vi "FFT Co-processor (FPGA) 6592R.vi"() -> ()   [LabVIEW 2014]
doc: "Data From Host Loop:\nThe FPGA target recieves a signal from the host from the Host-to-FPGA DMA FIFO and stores that data in the FIFO IN target-scoped FIFO. FIFO IN will not be written to if there is no information being read from the host and the Host-to-FPGA FIFO has timed out. The loop will stop if the user presses the stop control button or if the FIFO IN times out and data transfer from the host to the target is complete.\n\nFFT Processing Loop:\nWhen the FFT Express VI has signaled that it is ready for input, it will begin to read data from the FIFO IN target-scoped FIFO. The user has control over the output of the FFT Express VI. As the FFT VI computes the FFT it writes the resulting data to the FIFO OUT target-scoped VI when the FFT output is valid. The loop will stop if the user presses the stop control button or if the FIFO OUT times out and data transfer from the FFT VI to the FIFO is complete.\n\nData To Host Loop:\nFIFO OUT transfers data back to the host by writing the computed FFT signal data to the FPGA-to-Host DMA FIFO. When there is no data in FIFO OUT, it times out and stops writing to the host. At this point the data transfer is complete."
uses:
  <vilib>/Platform/TimedLoop/XDataNode/timing_clust.ctl
  <vilib>/Platform/TimedLoop/XDataNode/nitl_modes.ctl
  <vilib>/Platform/TimedLoop/XDataNode/wakeup.ctl
  <vilib>/rvi/Analysis/measure/FFT/simModelSupport/niFPGA FFT Streaming Sim Properties.ctl
  <vilib>/rvi/Analysis/measure/FFT/simModelSupport/niFPGA FFT Sim Stream Group Properties.ctl
  <vilib>/rvi/Analysis/measure/FFT/simModelSupport/niFPGA FFT Sim Types.ctl
  <vilib>/rvi/Analysis/measure/FFT/simModelSupport/niFpgaFFTSimArithmeticProperties.ctl
  <vilib>/rvi/Analysis/measure/FFT/simModelSupport/niFpgaFFTSimDfxp.ctl
  <vilib>/fxp/LVFixedPointQuantizationPolicyTypeDef.ctl
  <vilib>/rvi/Analysis/measure/FFT/XNode/niFpgaFFTButterflyDelays.ctl
  <vilib>/rvi/Analysis/measure/FFT/simModelSupport/niFPGA FFT Sim Properties.ctl
  <vilib>/rvi/Emulation/niFpgaSctlEmulationGetInTimedLoop.vi
  <vilib>/rvi/Emulation/niFpgaEmulationReportErrorSimple.vi
  <vilib>/rvi/Emulation/niFpgaGetClockAttributes.vi
  <vilib>/rvi/Emulation/niFpgaCriticalErrorInLSC.vi
  <vilib>/rvi/Emulation/niFpgaProcessEmulError.vi
  <vilib>/rvi/Emulation/niFpgaEmulationIsFPGAContextNoSignature.vi
  <vilib>/rvi/errors/niFpgaSetErrorForExecOnDevCompSimple.vi
  <vilib>/rvi/eio/common/nirviEmuReportErrorAndStop.vi
  <vilib>/rvi/DataTransferAndStorage/Container/Common/niFpgaContainerGetUniqueNameForEmu.vi
  <vilib>/rvi/FIFO/Fifo_Resource/nirvififoEmulationSetSize.vi
  <vilib>/rvi/FIFO/Fifo_Resource/nirviFifoEmulationQueueMgr.vi
  <instcachedir>/0/nirviFifoEmulationQueueMgr_E5CAEC123FF24DC58D834DCA3CDAA9B5.lvgen/nirviFifoEmulationQueueMgr_E5CAEC123FF24DC58D834DCA3CDAA9B5_002.vi
  <vilib>/Utility/error.llb/Clear Errors.vi
  <vilib>/rvi/FIFO/Fifo_Resource/nirvififoEmulationCreateLock.vi
  <vilib>/rvi/FIFO/Fifo_Resource/nirvififoEmulationObtainLock.vi
  <vilib>/rvi/FIFO/Fifo_Resource/nirvififoEmulationReleaseLock.vi
  <vilib>/rvi/occurrence/nirviWaitOnOccurrenceBase.vi
  <vilib>/rvi/errors/nirviReportUnexpectedCaseInternalError.vi
  <vilib>/rvi/errors/nirviReportUnexpectedCaseInternalError (U32).vi
  <vilib>/rvi/Analysis/measure/FFT/simModelSupport/niFpgaFFTSimModelStreamingCore.vi
  <vilib>/rvi/Analysis/measure/FFT/simModelSupport/niFpgaFFTSimModelCore.vi
  <vilib>/rvi/FIFO/Fifo_Resource/nirvififoEmulationDetermineInputValidOut.vi
  <vilib>/rvi/interface/RandomDataEmulation/niFpgaRandomDataHandleErrors.vi
  <vilib>/Platform/TimedLoop/XDataNode/XDataNode.xnode
  <vilib>/rvi/DataTransferAndStorage/Container/XNode/niFpgaContainer.xnode
  <vilib>/rvi/FIFO/Fifo_Resource/nirvififoEmulationRead.vi
  <vilib>/rvi/Analysis/measure/FFT/XNode/niFpgaFFT.xnode
  <vilib>/rvi/FIFO/Fifo_Resource/nirvififoEmulationWrite.vi
  <vilib>/rvi/interface/RandomDataEmulation/nirviRandomDataFpgaReadWriteTemplate.vi
  <vilib>/Platform/TimedLoop/XDataNode/XDNodeRunTimeDep.lvlib
panel:
  in  "FFT Size":i16=8192
  out "FFT Out":i32
  out "FIFO In (loop 2)":i32
  out "FIFO In":i32
  out "Host to FPGA":i32
  in  "stop":bool
  # "This FPGA VI continuously receives data from the host, performs a 1 kByte FFT, and then transfers the FFT results back to the host.  The input data type for the FFT is a 16-bit fixed point number with 8 bits of integer precision."
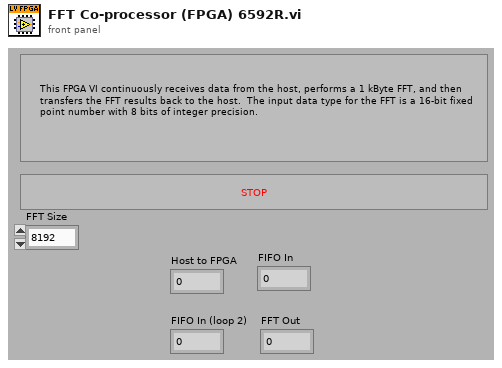
[diagram p1: front panel]
types:
  T1 = typedef "XDNodeRunTimeDep.lvlib/timing_clust.ctl" = cluster{"Expected End [f-1]":u64, "Actual End [f-1]":u64, "Finished Late? [f-1]":bool, "Expected End [i-1]":u64, "Actual End [i-1]":u64, "Finished Late? [i-1]":bool, "Expected Start [i]":u64, "Actual Start [i]":u64, "Expected Start [f]":u64, "Actual Start [f]":u64, "Source Name":string, "Structure Name":string, "Period":i64, "Deadline":i64, "Offset":i64, "Start":i64, "Priority":i32, "Timeout":i32, "Mode":T2, "Wakeup Reason":T3, "Error":errorcluster, "Source Type":string, "Secondary Source Type":string, "Global End Time":u64, "Global Start Time":u64, "Frame Duration":u64, "Iteration Duration":u64, "Assigned CPU":i32, "I/O Scan Engine Mode":u32}
  T2 = typedef "XDNodeRunTimeDep.lvlib/nitl_modes.ctl" = enum32{"No Change", "Process missed periods, maintain original phase", "Discard missed periods, maintain original phase", "Process missed periods, ignore original phase", "Discard missed periods, ignore original phase"}
  T3 = typedef "XDNodeRunTimeDep.lvlib/wakeup.ctl" = enum32{"Normal", "Aborted", "Asynchronous wakeup", "Timing source error", "Timed loop error", "Timeout"}
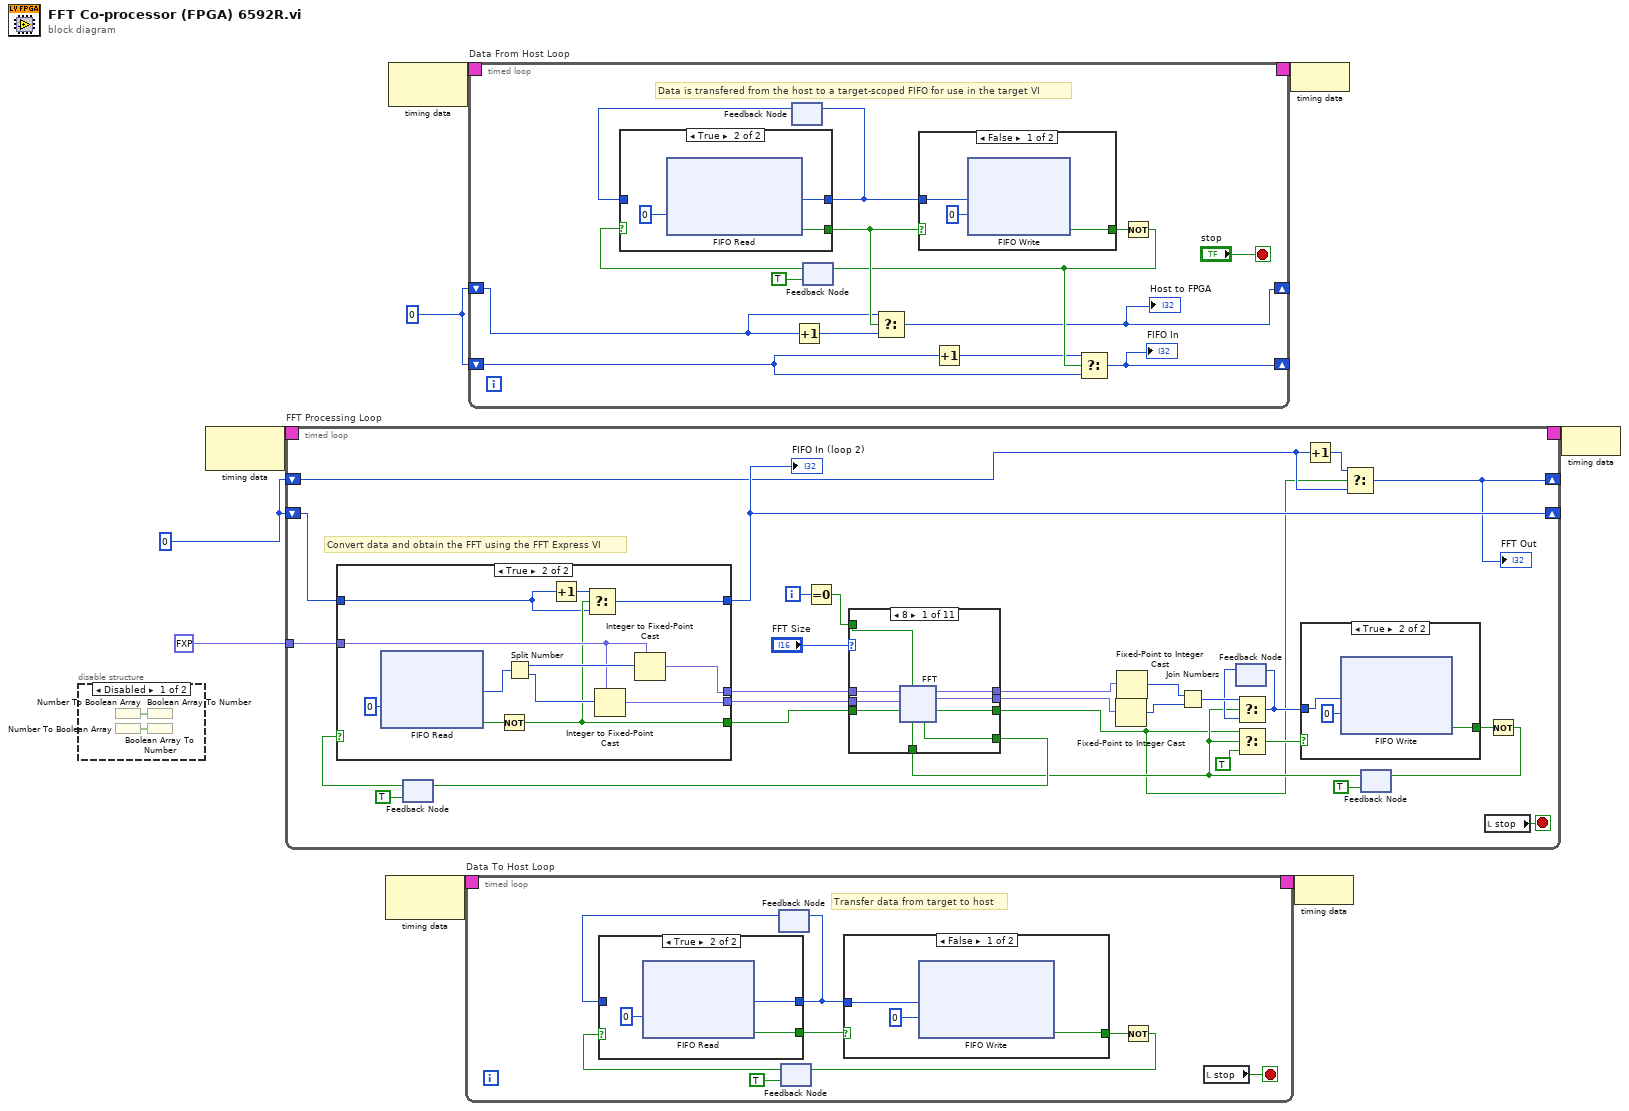
[diagram p0: block diagram]
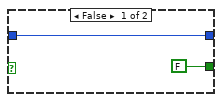
[diagram p3: hidden frame]
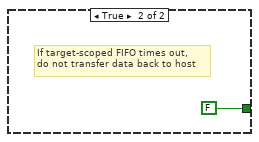
[diagram p4: hidden frame]
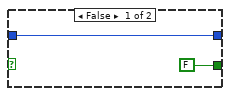
[diagram p5: hidden frame]
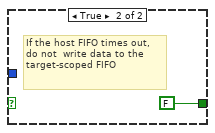
[diagram p6: hidden frame]
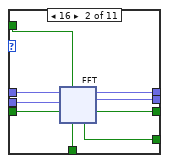
[diagram p7: hidden frame]
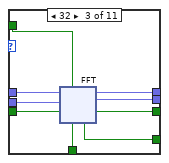
[diagram p8: hidden frame]
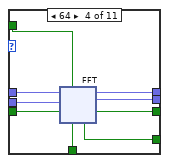
[diagram p9: hidden frame]
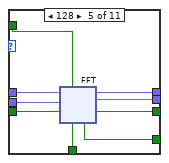
[diagram p10: hidden frame]
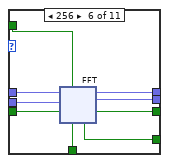
[diagram p11: hidden frame]
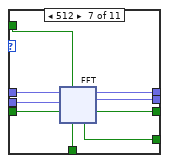
[diagram p12: hidden frame]
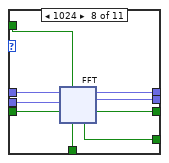
[diagram p13: hidden frame]
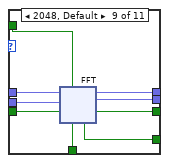
[diagram p14: hidden frame]
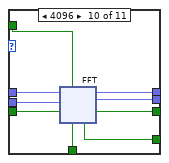
[diagram p15: hidden frame]
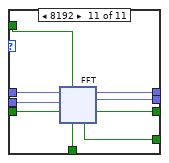
[diagram p16: hidden frame]
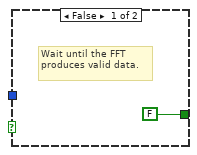
[diagram p17: hidden frame]
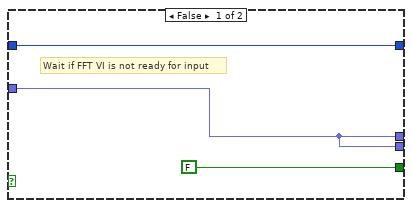
[diagram p18: hidden frame]
diagram:
  w1 = 0 ("Timeout")
  w2 = 0 ("Timeout")
  n1 = disable-structure shown="Disabled" {
    frame Disabled {
      n2 = Number To Boolean Array() -> (Boolean array=w11:bool[])  [unwired: 1 in]
      n3 = Number To Boolean Array() -> (Boolean array=w10:bool[])  [unwired: 1 in]
      n4 = Boolean Array To Number(Boolean array=w11) -> ()  [unwired: 1 out]
      n5 = Boolean Array To Number(Boolean array=w10) -> ()  [unwired: 1 out]
    }
    frame Enabled {
    }
  }
  n6 = node-c288() -> (w9:T1)  [unwired: 1 out]
  n7 = timed-loop "FFT Processing Loop" {
    timing: w9 -> [_]
    timing-out: [_] -> w8
    tunnel: fxp<+/-,24,0> 0.0 ("real data in") -> [w25]
    shift-right: [w23] -> _
    shift-left: w1 -> [w24]
    shift-right: [w20] -> _
    shift-left: w1 -> [w21]
    i -> [w39]
    stop <- w36 stop-if-true
    # "Convert data and obtain the FFT using the FFT Express VI"
    n8 = feedback #1(TRUE ("ready for data")) -> (w41:bool)
    n9 = case shown="True" w41 {
      tunnel: [FALSE w437] -> w26
      tunnel: [w432 w440] -> w18
      tunnel: w25 -> [w432 w439]
      tunnel: [w432 w438] -> w17
      tunnel: w24 -> [w431 w435]
      tunnel: [w431 w434] -> w23
      frame False {
        # "Wait if FFT VI is not ready for input"
      }
      frame True {
        n10 = xnode ("FIFO Read")("Timeout"=0) -> ("Element"=w443:u64, "Timed Out?"=w445:bool)  [unwired: 1 in, 1 out]
        n11 = Not(x=w445) -> (.not. x?=w437:bool)
        n12 = Split Number(x=w443) -> (hi(x)=w442:u32, lo(x)=w441:u32)
        n13 = Increment(x=w435) -> (x+1=w436:i32)
        n14 = Select(t=w436, s=w437, f=w435) -> (s? t:f=w434:i32)
        n15 = Integer to Fixed-Point Cast(fixed-point type=w439, integer=w441) -> (fixed-point=w438:fxp<+/-,24,0>)
        n16 = Integer to Fixed-Point Cast(fixed-point type=w439, integer=w442) -> (fixed-point=w440:fxp<+/-,24,0>)
      }
    }
    "FIFO In (loop 2)" <- w23
    n17 = Equal To 0?(x=w39) -> (x = 0?=w38:bool)
    n18 = feedback #2() -> (w31:u64)  [unwired: 1 out]
    n19 = Increment(x=w21) -> (x+1=w22:i32)
    n20 = feedback #3(TRUE ("ready for data")) -> (w28:bool)
    n21 = case shown="8" "FFT Size" {
      tunnel: w38 -> [w50 w85 w120 w155 w190 w225 w260 w295 w330 w365 w400]
      tunnel: [w49 w84 w119 w154 w189 w224 w259 w294 w329 w364 w399] -> w37
      tunnel: w28 -> [w48 w83 w118 w153 w188 w223 w258 w293 w328 w363 w398]
      tunnel: w26 -> [w47 w82 w117 w152 w187 w222 w257 w292 w327 w362 w397]
      tunnel: [w46 w81 w116 w151 w186 w221 w256 w291 w326 w361 w396] -> w19
      tunnel: w18 -> [w45 w80 w115 w150 w185 w220 w255 w290 w325 w360 w395]
      tunnel: w17 -> [w44 w79 w114 w149 w184 w219 w254 w289 w324 w359 w394]
      tunnel: [w43 w78 w113 w148 w183 w218 w253 w288 w323 w358 w393] -> w16
      tunnel: [w42 w77 w112 w147 w182 w217 w252 w287 w322 w357 w392] -> w15
      frame 8 {
        n22 = xnode "FFT"("real data in"=w45, "reset"=w50, "imaginary data in"=w44, "input valid"=w47, "ready for output"=w48) -> ("ready for input"=w49:bool, "real data out"=w43:fxp<+/-,28,4>, "imaginary data out"=w42:fxp<+/-,28,4>, "output valid"=w46:bool)  [unwired: 1 out]
      }
      frame 16 {
        n23 = xnode "FFT"("real data in"=w80, "reset"=w85, "imaginary data in"=w79, "input valid"=w82, "ready for output"=w83) -> ("ready for input"=w84:bool, "real data out"=w78:fxp<+/-,29,5>, "imaginary data out"=w77:fxp<+/-,29,5>, "output valid"=w81:bool)  [unwired: 1 out]
      }
      frame 32 {
        n24 = xnode "FFT"("real data in"=w115, "reset"=w120, "imaginary data in"=w114, "input valid"=w117, "ready for output"=w118) -> ("ready for input"=w119:bool, "real data out"=w113:fxp<+/-,30,6>, "imaginary data out"=w112:fxp<+/-,30,6>, "output valid"=w116:bool)  [unwired: 1 out]
      }
      frame 64 {
        n25 = xnode "FFT"("real data in"=w150, "reset"=w155, "imaginary data in"=w149, "input valid"=w152, "ready for output"=w153) -> ("ready for input"=w154:bool, "real data out"=w148:fxp<+/-,31,7>, "imaginary data out"=w147:fxp<+/-,31,7>, "output valid"=w151:bool)  [unwired: 1 out]
      }
      frame 128 {
        n26 = xnode "FFT"("real data in"=w185, "reset"=w190, "imaginary data in"=w184, "input valid"=w187, "ready for output"=w188) -> ("ready for input"=w189:bool, "real data out"=w183:fxp<+/-,32,8>, "imaginary data out"=w182:fxp<+/-,32,8>, "output valid"=w186:bool)  [unwired: 1 out]
      }
      frame 256 {
        n27 = xnode "FFT"("real data in"=w220, "reset"=w225, "imaginary data in"=w219, "input valid"=w222, "ready for output"=w223) -> ("ready for input"=w224:bool, "real data out"=w218:fxp<+/-,32,9>, "imaginary data out"=w217:fxp<+/-,32,9>, "output valid"=w221:bool)  [unwired: 1 out]
      }
      frame 512 {
        n28 = xnode "FFT"("real data in"=w255, "reset"=w260, "imaginary data in"=w254, "input valid"=w257, "ready for output"=w258) -> ("ready for input"=w259:bool, "real data out"=w253:fxp<+/-,32,10>, "imaginary data out"=w252:fxp<+/-,32,10>, "output valid"=w256:bool)  [unwired: 1 out]
      }
      frame 1024 {
        n29 = xnode "FFT"("real data in"=w290, "reset"=w295, "imaginary data in"=w289, "input valid"=w292, "ready for output"=w293) -> ("ready for input"=w294:bool, "real data out"=w288:fxp<+/-,32,11>, "imaginary data out"=w287:fxp<+/-,32,11>, "output valid"=w291:bool)  [unwired: 1 out]
      }
      frame 2048, Default {
        n30 = xnode "FFT"("real data in"=w325, "reset"=w330, "imaginary data in"=w324, "input valid"=w327, "ready for output"=w328) -> ("ready for input"=w329:bool, "real data out"=w323:fxp<+/-,32,12>, "imaginary data out"=w322:fxp<+/-,32,12>, "output valid"=w326:bool)  [unwired: 1 out]
      }
      frame 4096 {
        n31 = xnode "FFT"("real data in"=w360, "reset"=w365, "imaginary data in"=w359, "input valid"=w362, "ready for output"=w363) -> ("ready for input"=w364:bool, "real data out"=w358:fxp<+/-,32,13>, "imaginary data out"=w357:fxp<+/-,32,13>, "output valid"=w361:bool)  [unwired: 1 out]
      }
      frame 8192 {
        n32 = xnode "FFT"("real data in"=w395, "reset"=w400, "imaginary data in"=w394, "input valid"=w397, "ready for output"=w398) -> ("ready for input"=w399:bool, "real data out"=w393:fxp<+/-,32,14>, "imaginary data out"=w392:fxp<+/-,32,14>, "output valid"=w396:bool)  [unwired: 1 out]
      }
    }
    n33 = feedback-in #1(w37) -> ()
    n34 = Fixed-Point to Integer Cast(1:w15) -> (0:w14:i64)
    n35 = Fixed-Point to Integer Cast(1:w16) -> (0:w13:i64)
    n36 = Join Numbers(hi=w13, lo=w14) -> ((hi.lo)=w32:u64)
    n37 = Select(t=w32, s=w28, f=w31) -> (s? t:f=w30:u64)
    n38 = feedback-in #2(w30) -> ()
    n39 = Select(t=w19, s=w28, f=TRUE) -> (s? t:f=w29:bool)
    n40 = case shown="True" w29 {
      tunnel: [FALSE ("Timed Out?") w429] -> w35
      tunnel: w30 -> [_ w428]
      frame False {
        # "Wait until the FFT produces valid data."
      }
      frame True {
        n41 = xnode ("FIFO Write")("Element"=w428, "Timeout"=0) -> ("Timed Out?"=w429:bool)  [unwired: 1 in, 1 out]
      }
    }
    n42 = Select(t=w22, s=w19, f=w21) -> (s? t:f=w20:i32)
    "FFT Out" <- w20
    n43 = local read "stop"() -> (w36:bool)
    n44 = Not(x=w35) -> (.not. x?=w33:bool)
    n45 = feedback-in #3(w33) -> ()
  }
  n46 = node-c288() -> (w5:T1)  [unwired: 1 out]
  n47 = node-c288() -> (w7:T1)  [unwired: 1 out]
  n48 = timed-loop "Data To Host Loop" {
    timing: w5 -> [_]
    timing-out: [_] -> w4
    stop <- w454 stop-if-true
    # "Transfer data from target to host"
    n49 = feedback #4() -> (w452:u64)  [unwired: 1 out]
    n50 = feedback #5(TRUE) -> (w448:bool)
    n51 = case shown="True" w448 {
      tunnel: [FALSE ("Timed Out?") w459] -> w455
      tunnel: [w457 w458] -> w453
      tunnel: w452 -> [w457 _]
      frame False {
      }
      frame True {
        n52 = xnode ("FIFO Read")("Timeout"=0) -> ("Element"=w458:u64, "Timed Out?"=w459:bool)  [unwired: 1 in, 1 out]
      }
    }
    n53 = feedback-in #4(w453) -> ()
    n54 = case shown="False" w455 {
      tunnel: [w461 FALSE ("Timed Out?")] -> w451
      tunnel: w453 -> [w463 _]
      frame False {
        n55 = xnode ("FIFO Write")("Element"=w463, "Timeout"=0) -> ("Timed Out?"=w461:bool)  [unwired: 1 in, 1 out]
      }
      frame True {
        # "If target-scoped FIFO times out, \ndo not transfer data back to host"
      }
    }
    n56 = Not(x=w451) -> (.not. x?=w449:bool)
    n57 = feedback-in #5(w449) -> ()
    n58 = local read "stop"() -> (w454:bool)
  }
  n59 = timed-loop "Data From Host Loop" {
    timing: w7 -> [_]
    timing-out: [_] -> w6
    shift-right: [w472] -> _
    shift-left: w2 -> [w470]
    shift-right: [w471] -> _
    shift-left: w2 -> [w468]
    stop <- "stop" stop-if-true
    # "Data is transfered from the host to a target-scoped FIFO for use in the target VI"
    n60 = feedback #6() -> (w475:u64)  [unwired: 1 out]
    n61 = Increment(x=w470) -> (x+1=w469:i32)
    n62 = feedback #7(TRUE) -> (w477:bool)
    n63 = case shown="True" w477 {
      tunnel: [FALSE ("Timed Out?") w485] -> w474
      tunnel: [w482 w483] -> w476
      tunnel: w475 -> [w482 _]
      frame False {
      }
      frame True {
        n64 = xnode ("FIFO Read")("Timeout"=0) -> ("Element"=w483:u64, "Timed Out?"=w485:bool)  [unwired: 1 in, 1 out]
      }
    }
    n65 = feedback-in #6(w476) -> ()
    n66 = Select(t=w470, s=w474, f=w469) -> (s? t:f=w472:i32)
    "Host to FPGA" <- w472
    n67 = case shown="False" w474 {
      tunnel: w476 -> [w487 _]
      tunnel: [w486 FALSE ("Timed Out?")] -> w479
      frame False {
        n68 = xnode ("FIFO Write")("Element"=w487, "Timeout"=0) -> ("Timed Out?"=w486:bool)  [unwired: 1 in, 1 out]
      }
      frame True {
        # "If the host FIFO times out, do not  write data to the target-scoped FIFO"
      }
    }
    n69 = Increment(x=w468) -> (x+1=w467:i32)
    n70 = Not(x=w479) -> (.not. x?=w473:bool)
    n71 = feedback-in #7(w473) -> ()
    n72 = Select(t=w467, s=w473, f=w468) -> (s? t:f=w471:i32)
    "FIFO In" <- w471
  }
  n73 = node-c288(w6) -> ()
  n74 = node-c288(w4) -> ()
  n75 = node-c288(w8) -> ()
